vi "IHL_Inspect-Stop Helper.vi"(8 "error in (no error)":errorcluster, 10 "Inspect Helper Loop Data":T1={"IHL State"=enum."Init", "Timeout"=0, "Loop Count"=0, "Start Sample No."=0, "No. Samples"=0, "Collecting Data"=FALSE, "Scan Complete"=FALSE, "Inspect Status "={"Ready"=FALSE, "Inspecting"=FALSE, "Cancel"=FALSE}, "Status"=0, "Encoder Count"=0, "PosToStartScan"=50800, "ScanLength"=50800, "MaxSamples"=50800, "PosToEndScan"=0, "data value reference"=refnum, "Block Cnt notifier out"=refnum, "EventLog"=refnum}, 11 "Message Queue in":refnum<class "Delacor_lib_QMH_Message Queue.lvclass">) -> (0 "error out":errorcluster, 2 "Inspect Helper Loop Data out":T1={"IHL State"=enum."Init", "Timeout"=0, "Loop Count"=0, "Start Sample No."=0, "No. Samples"=0, "Collecting Data"=FALSE, "Scan Complete"=FALSE, "Inspect Status "={"Ready"=FALSE, "Inspecting"=FALSE, "Cancel"=FALSE}, "Status"=0, "Encoder Count"=0, "PosToStartScan"=50800, "ScanLength"=50800, "MaxSamples"=50800, "PosToEndScan"=0, "data value reference"=refnum, "Block Cnt notifier out"=refnum, "EventLog"=refnum}, 3 "State String":string="IHL:Timeout: Inspect: STOP")   [LabVIEW 2015, in "Tool Module.lvlib"]
uses:
  Tool Module.lvlib
  <vilib>/Delacor/Delacor QMH/Libraries/Message Queue_class/Delacor_lib_QMH_Message Queue.lvclass
  _IHL Data Cluster--typedef.ctl
  QC-X App/Libraries/Event Logger Library/Event Log/EventLog.lvclass
  _IHL SM Enum--typedef.ctl
  _IHL Status Update Cluster--typedef.ctl
  <vilib>/Delacor/Delacor QMH/Libraries/Message Queue_class/Delacor_lib_QMH_Message Queue.lvclass/Delacor_lib_QMH_Message Queue.ctl
  <vilib>/Delacor/Delacor QMH/Libraries/Message Queue_class/Delacor_lib_QMH_Enqueue Message (Array).vi
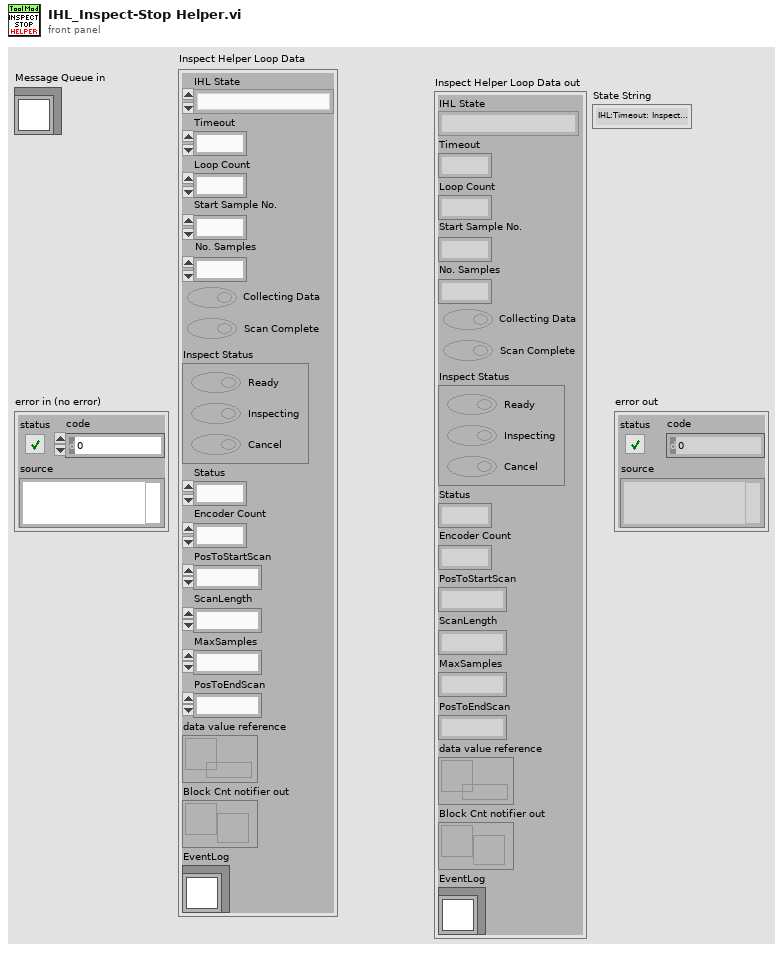
[diagram p1: front panel]
types:
  T1 = typedef "Tool Module.lvlib/_IHL Data Cluster--typedef.ctl" = cluster{"IHL State":T2, "Timeout":i32, "Loop Count":i32, "Start Sample No.":u32, "No. Samples":i32, "Collecting Data":bool, "Scan Complete":bool, "Inspect Status ":T3, "Status":u16, "Encoder Count":i32, "PosToStartScan":i32, "ScanLength":i32, "MaxSamples":i32, "PosToEndScan":i32, "data value reference":refnum<data-value>, "Block Cnt notifier out":refnum<notifier>, "EventLog":refnum<class "EventLog.lvclass">}
  T2 = typedef "Tool Module.lvlib/_IHL SM Enum--typedef.ctl" = enum16{"Init", "Set Motion Speed", "Move To Scan Start", "Wait for Motion Out", "Wait for Start Pos", "Inspect: START", "Wait for Motion IN", "Wait for Inspect Range", "Inspecting", "Inspect: STOP"}
  T3 = typedef "Tool Module.lvlib/_IHL Status Update Cluster--typedef.ctl" = cluster{"Ready":bool, "Inspecting":bool, "Cancel":bool}
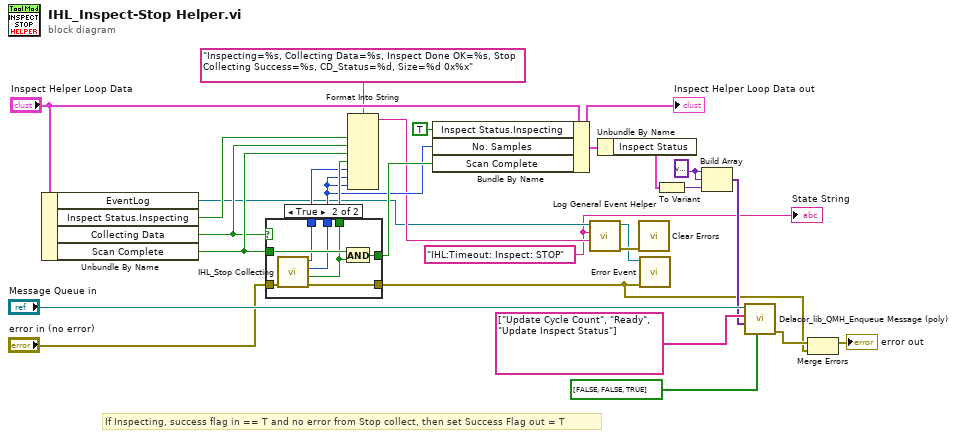
[diagram p0: block diagram]
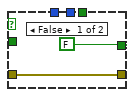
[diagram p2: hidden frame]
diagram:
  w12 = variant ("Message Data")
  w2 = "IHL:Timeout: Inspect: STOP"
  # "If Inspecting, success flag in == T and no error from Stop collect, then set Success Flag out = T"
  n1 = Unbundle By Name("Inspect Helper Loop Data") -> ("EventLog"=w4:refnum<class "EventLog.lvclass">, "Inspect Status.Inspecting"=w17:bool, "Collecting Data"=w5:bool, "Scan Complete"=w18:bool)
  n2 = case shown="True" w5 {
    tunnel: [w28 w36] -> w1
    tunnel: [FALSE w31] -> w25
    tunnel: w18 -> [_ w35]
    tunnel: [_ w34] -> w24
    tunnel: [_ w33] -> w19
    tunnel: [_ w32] -> w23
    tunnel: "error in (no error)" -> [w28 w30]
    frame False {
    }
    frame True {
      n3 = call "IHL_Stop Collecting.vi"("error in (no error)"=w30) -> ("error out"=w36:errorcluster, "Success"=w34:bool, "Array Size"=w32:u32, "CD Status"=w33:i32)  [unwired: 7 in]
      n4 = And(x=w35, y=w34) -> (x .and. y?=w31:bool)
    }
  }
  n5 = Format Into String(format string="Inspecting=%s, Collecting Data=%s, Inspect Done OK=%s, Stop Collecting Success=%s, CD_Status=%d, Size=%d 0x%x", w17, w5, w18, w24, w19, w23, w23) -> (resulting string=w21:string)  [unwired: 2 in, 1 out]
  n6 = Bundle By Name(cluster="Inspect Helper Loop Data", "Inspect Status.Inspecting"=TRUE ("Inspect Status .Inspecting"), "No. Samples"=w23, "Scan Complete"=w25) -> (w11:T1)
  "Inspect Helper Loop Data out" <- w11
  n7 = call "Log General Event Helper.vi"("Payload"=w21, "State Info"=w2, "EventLog in"=w4) -> ("error out"=w27:errorcluster, "EventLog out"=w3:refnum<class "EventLog.lvclass">)  [unwired: 7 in]
  n8 = Unbundle By Name(w11) -> ("Inspect Status"=w7:T3)
  n9 = call <vilib>:"Clear Errors.vi"("error in (no error)"=w27) -> ()  [unwired: 5 in, 2 out]
  n10 = call "Error Event.vi"("error in (no error)"=w1, "EventLog ref"=w3) -> ()  [unwired: 8 in, 2 out]
  n11 = To Variant(anything=w7) -> (Variant=w6:variant)
  n12 = Build Array(w12, w12, w6) -> (w13:variant[])
  n13 = call-poly <vilib>:"Delacor_lib_QMH_Enqueue Message (poly).vi"("Priority Message? Array"=bool[] [FALSE, FALSE, TRUE], "Message Data Array"=w13, "Message Array"=string[] ["Update Cycle Count", "Ready", "Update Inspect Status"] ("Message"), "Message Queue in"="Message Queue in") -> ("error out"=w9:errorcluster)  [unwired: 6 in, 1 out]
  n14 = Merge Errors(w9, w1) -> (→"error out":errorcluster)
  "State String" <- w2
